vi "Dashboard Main.vi"() -> ()   [LabVIEW 2014]
uses:
  <vilib>/event_ctls.llb/eventvkey.ctl
  <vilib>/Rock Robotics/WPI/Dashboard/WPI_DashboardLogging Global.vi
  <vilib>/Rock Robotics/Network Tables/SD Write Number.vi
  <vilib>/Rock Robotics/Network Tables/SD Write Boolean.vi
  <vilib>/Rock Robotics/Network Tables/SD Read Number.vi
  <vilib>/Rock Robotics/Network Tables/SD Read Boolean.vi
  <vilib>/Rock Robotics/Network Tables/SD Write String.vi
  <vilib>/Utility/config.llb/Write Key (String).vi
  <vilib>/Utility/config.llb/Write Key (I32).vi
  <vilib>/Utility/config.llb/NI_LVConfig.lvlib
panel:
  in  "TCP":refnum<k5>
  in  "Rec Mode":enum32{"Stop", "Record", "Playback"}(radio)
  in  "Vision":u16(ring) items=["Camera Off", "USB Camera SW", "USB Camera HW", "IP Camera"]
  out "Camera IP":string
  out "Image Message":string="Timeout in Camera Communications"
  in  "Dashboard Tab":T1(tab)
  out "Lower Sensor":bool
  out "Middle Sensor":bool
  out "Overide":bool=TRUE
  out "Lift Saftey":bool
  out "Top Sensor":bool
  out "Bottom Sensor":bool
  out "?":bool
  in  "Motor Saftey":bool=TRUE
  in  "Camera Settings":T2={"Frame Rate"=30, "Compression"=30, "Size"=1} {"Frame Rate" scale=1.0..30.0; "Size" items=["640x480", "320x240", "160x120"]}
  out "Gyro":dbl(knob) scale=0.0..360.0
  out "Mode":T3(ring)=enum."Auto Disabled"
  in  "DB Camera Config":bool
  out "fps":dbl format="%#.1g"
  out "Mbps":dbl format="%#.1g"
  out "Mbps 2":bool
  in  "DB/String 9":string
  in  "DB/String 8":string
  in  "DB/String 7":string
  in  "DB/String 6":string
  in  "DB/String 5":string
  in  "DB/String 4":string
  in  "DB/String 3":string
  in  "DB/String 2":string
  in  "DB/String 1":string
  in  "DB/String 0":string
  in  "DB/Slider 0":dbl(slide) scale=0.0..5.0
  in  "DB/Slider 1":dbl(slide) scale=0.0..5.0
  in  "DB/Slider 2":dbl(slide) scale=0.0..5.0
  in  "DB/Slider 3":dbl(slide) scale=0.0..5.0
  out "DB/LED 3":bool
  out "DB/LED 2":bool
  out "DB/LED 1":bool
  out "DB/LED 0":bool
  in  "DB/Button 3":bool
  in  "DB/Button 2":bool
  in  "DB/Button 1":bool
  in  "DB/Button 0":bool caption="New Name"
  in  "Test Slider":dbl(slide) scale=0.0..100.0 scale format="%#_3g"
  in  "On/Off":bool caption="Solenoid"
  in  "Test Name":u16(ring) items=["Select the test to run...", "Example Test", "-------------------------------", "List of tests is built in robot code.", "Replace with your own automated tests."]
  in  "Test Tree":string(tree)
  in  "Motor":cluster{"Value":dbl, "Enable":bool} {"Value" scale=-1.0..1.0 scale format="%#_3g"}
  out "Progress":T4 {"Test Progress" scale=0.0..100.0}
  in  "Rev/Fwd":cluster{"Forward":bool, "Reverse":bool}
  in  "Test Ring":u16(ring) items=["Monochrome", "Color"]
  in  "Listbox":i32(listbox)
  in  "Listbox 2":i32(listbox)=15
  in  "Autonomous Program":i32(listbox)
  in  "Test System Select":enum32{"Motors", "Pneumatics"}(tab)
  in  "Test Motor Mode Select":enum32{"Encoder Mode", "Manual Mode"}(tab)
  in  "?":bool
  in  "Motor Power":dbl(knob) scale=0.0..1.0
  out "?":bool=TRUE
  out "Encoder Feedback":dbl
  in  "Encoder Setpoint":dbl
  out "Encoder RPM":dbl
  in  "?":dbl(knob) scale=-1.0..1.0
  in  "Test Action":string(combo)="Disabled"
  out "?":string="Click the top button to toggle compressor state.\nThe green button indicates if the compressor is running. If the pressure in the system is above 100psi the compressor will turn off."
  out "?":bool
  in  "?":bool
  in  "?":bool
  in  "Solenoid Action":string(combo)="Disabled"
  out "Tree":string(tree)
  out "Camera Image":T5(plugin-control)
  out "Boolean":bool
  # "Top"
  # "Middle"
  # "Lift Saftey"
  # "Lower"
  # "Bottom"
  # "Overide"
  # "This tab is a great place for autonomous settings and robot-specific values.\nPlace controls and indicators inside this tab and match name to\nDashboard Variables on robot. You can also delete this comment."
  # "Select a system to test."
  # "Type in encoder setpoint (Ticks). Then increase the power slowly.  Encoder feedback is the traveled distance.\nThe motor should stop when staus button is green. Press reset to reset encoder."
  # "Simply drag the needle to change motor power. Motor RPM is below."
  # "Pick an action an click the button above. Double acting solenoids are automatically changed."
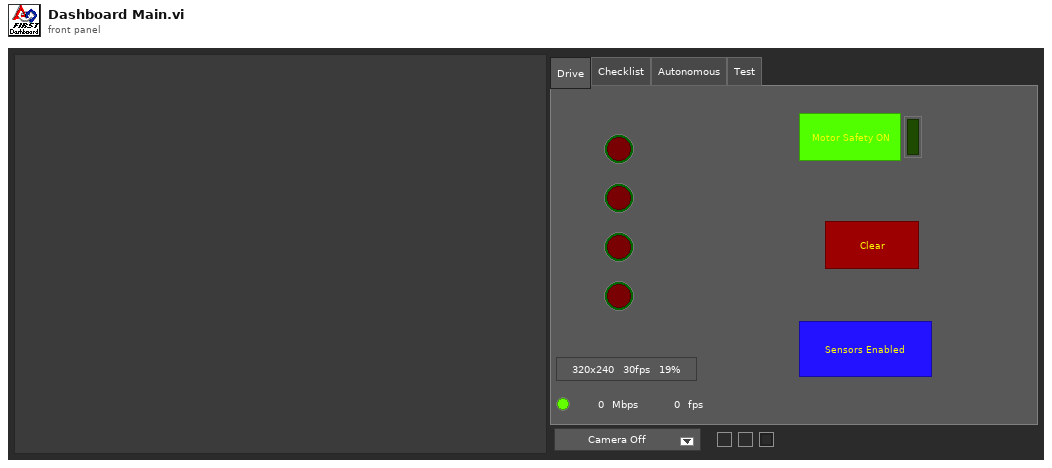
[diagram p1: front panel]
types:
  T1 = enum32{"Drive", "Basic", "Custom", "Test Var", "ChecklistOLD", "Checklist", "Autonomous", "Test", "Variables"}
  T2 = cluster{"Frame Rate":i32, "Compression":i32, "Size":u16}
  T3 = enum8{"Tele-Op Disabled", "Tele-Op Enabled", "Auto Disabled", "Auto Enabled", "Test Disabled", "Test Enabled", "Disconnected", "No Code", "E-Stop"}
  T4 = cluster{"Test Progress":u8, "Test Progress Text":string}
  T5 = typedef "IMAQ Image.ctl" = refnum<image>
  T6 = enum32{"Drive", "Basic", "Custom", "Test", "Checklist", "Variables"}
  T7 = typedef "Image Type" = u32
  T8 = cluster{"Camera Image":refnum<vi>, "Dashboard Tab":refnum<vi>, "Boolean":refnum<vi>, "Vision":refnum<vi>, "Rec Mode":refnum<vi>, "Test Slider":refnum<vi>, "On/Off ":refnum<vi>, "Test Ring":refnum<vi>, "Rev/Fwd":refnum<vi>, "Test Name":refnum<vi>, "Motor":refnum<vi>, "Progress":refnum<vi>, "CheckList":refnum<vi>, "Tree":refnum<vi>, "Test Tree":refnum<vi>}
  T9 = cluster{"Error Strings":string, "Disable Counts":cluster{u16, u16}, "Rail Faults":cluster{u16, u16, u16}, "Robot IP":string, "DB Mode":u8, "Event Info":cluster{"Name":string, "Type":u8, "Number":u16, "Replay":u8}, "Camera Addr":string}
  T10 = cluster{"Storage":cluster{"Disk Free":u64, "RAM Block":u32, "RAM free":u32}, "CPU Utilization":cluster{"CPU % ISR":sgl, "CPU % Time Crit":sgl, "CPU % Timed Str":sgl, "CPU % High":sgl, "CPU % Above":sgl, "CPU % Normal":sgl, "CPU % Low":sgl}, "CAN":cluster{"% Bus Utilization":sgl, "Bus Off Cnt":u32, "TX_FIFO Full Cnt":u32, "Receive Error Cnt":u8, "Transmit Error Cnt":u8}, "HID":cluster{"HID Outputs":u32, "Rumble Low":u16, "Rumble High":u16}[]}
  T11 = cluster{"Status bits":cluster{"Test Mode":bool, "Autonomous":bool, "Enabled":bool, "Code Start":bool, "Brownout":bool, "Reserved 2":bool, "Reserved 3":bool, "E-Stop":bool}, "Code Trace":cluster{"Disabled":bool, "TeleOp":bool, "Auto":bool, "Test":bool}, "Controller Type":enum16{"unknown", "cRIO", "roboRio"}, "Code?":enum16{"unknown", "noCode", "code"}, "Battery V":dbl}
  T12 = cluster{"Control Bits":cluster{"TestMode":bool, "Autonomous":bool, "Enabled":bool, "FMS Present":bool, bool, bool, bool, "E-Stop":bool}, "Team Station ":u8, "Countdown":sgl, "Joystick Values":cluster{"Axes":dbl[], "Buttons":bool[], "POVs":i16[]}[]}
  T13 = typedef "NI_LVConfig.lvlib/Config Data RefNum.ctl" = refnum<k1>
  T14 = cluster{"Operation":enum16{"Update", "Clear"}, "Color Box":u32}[]
  T15 = typedef "eventvkey.ctl" = enum16{"ASCII", "Enter", "Return", "Shift", "Ctrl", "Alt", "Cmd", "Opt", "Caps", "NumLock", "Clear", "Break", "Up", "Down", "Left", "Right", "Insert", "Delete", "Home", "End", "PageUp", "PageDown", "Escape", "Help", "Pause", "ScrollLock", "F1", "F2", "F3", "F4", "F5", "F6", "F7", "F8", "F9", "F10", "F11", "F12", "F13", "F14", "F15", "F16", "F17", "F18", "F19", "F20", "F21", "F22", "F23", "F24", "Play", "VolumeUp", "VolumeDown", "Mute", "Two Byte Char"}
  T16 = cluster{"Image Size":bool, "Image Type":bool, "Pixel Value":bool, "ROI Information":bool, "Zoom Factor":bool}
  T17 = enum8{"Enabled", "Disabled", "Disabled and Grayed Out"}
  T18 = cluster{"Operation":enum16{"Update", "Clear"}, "Color Box":u32}
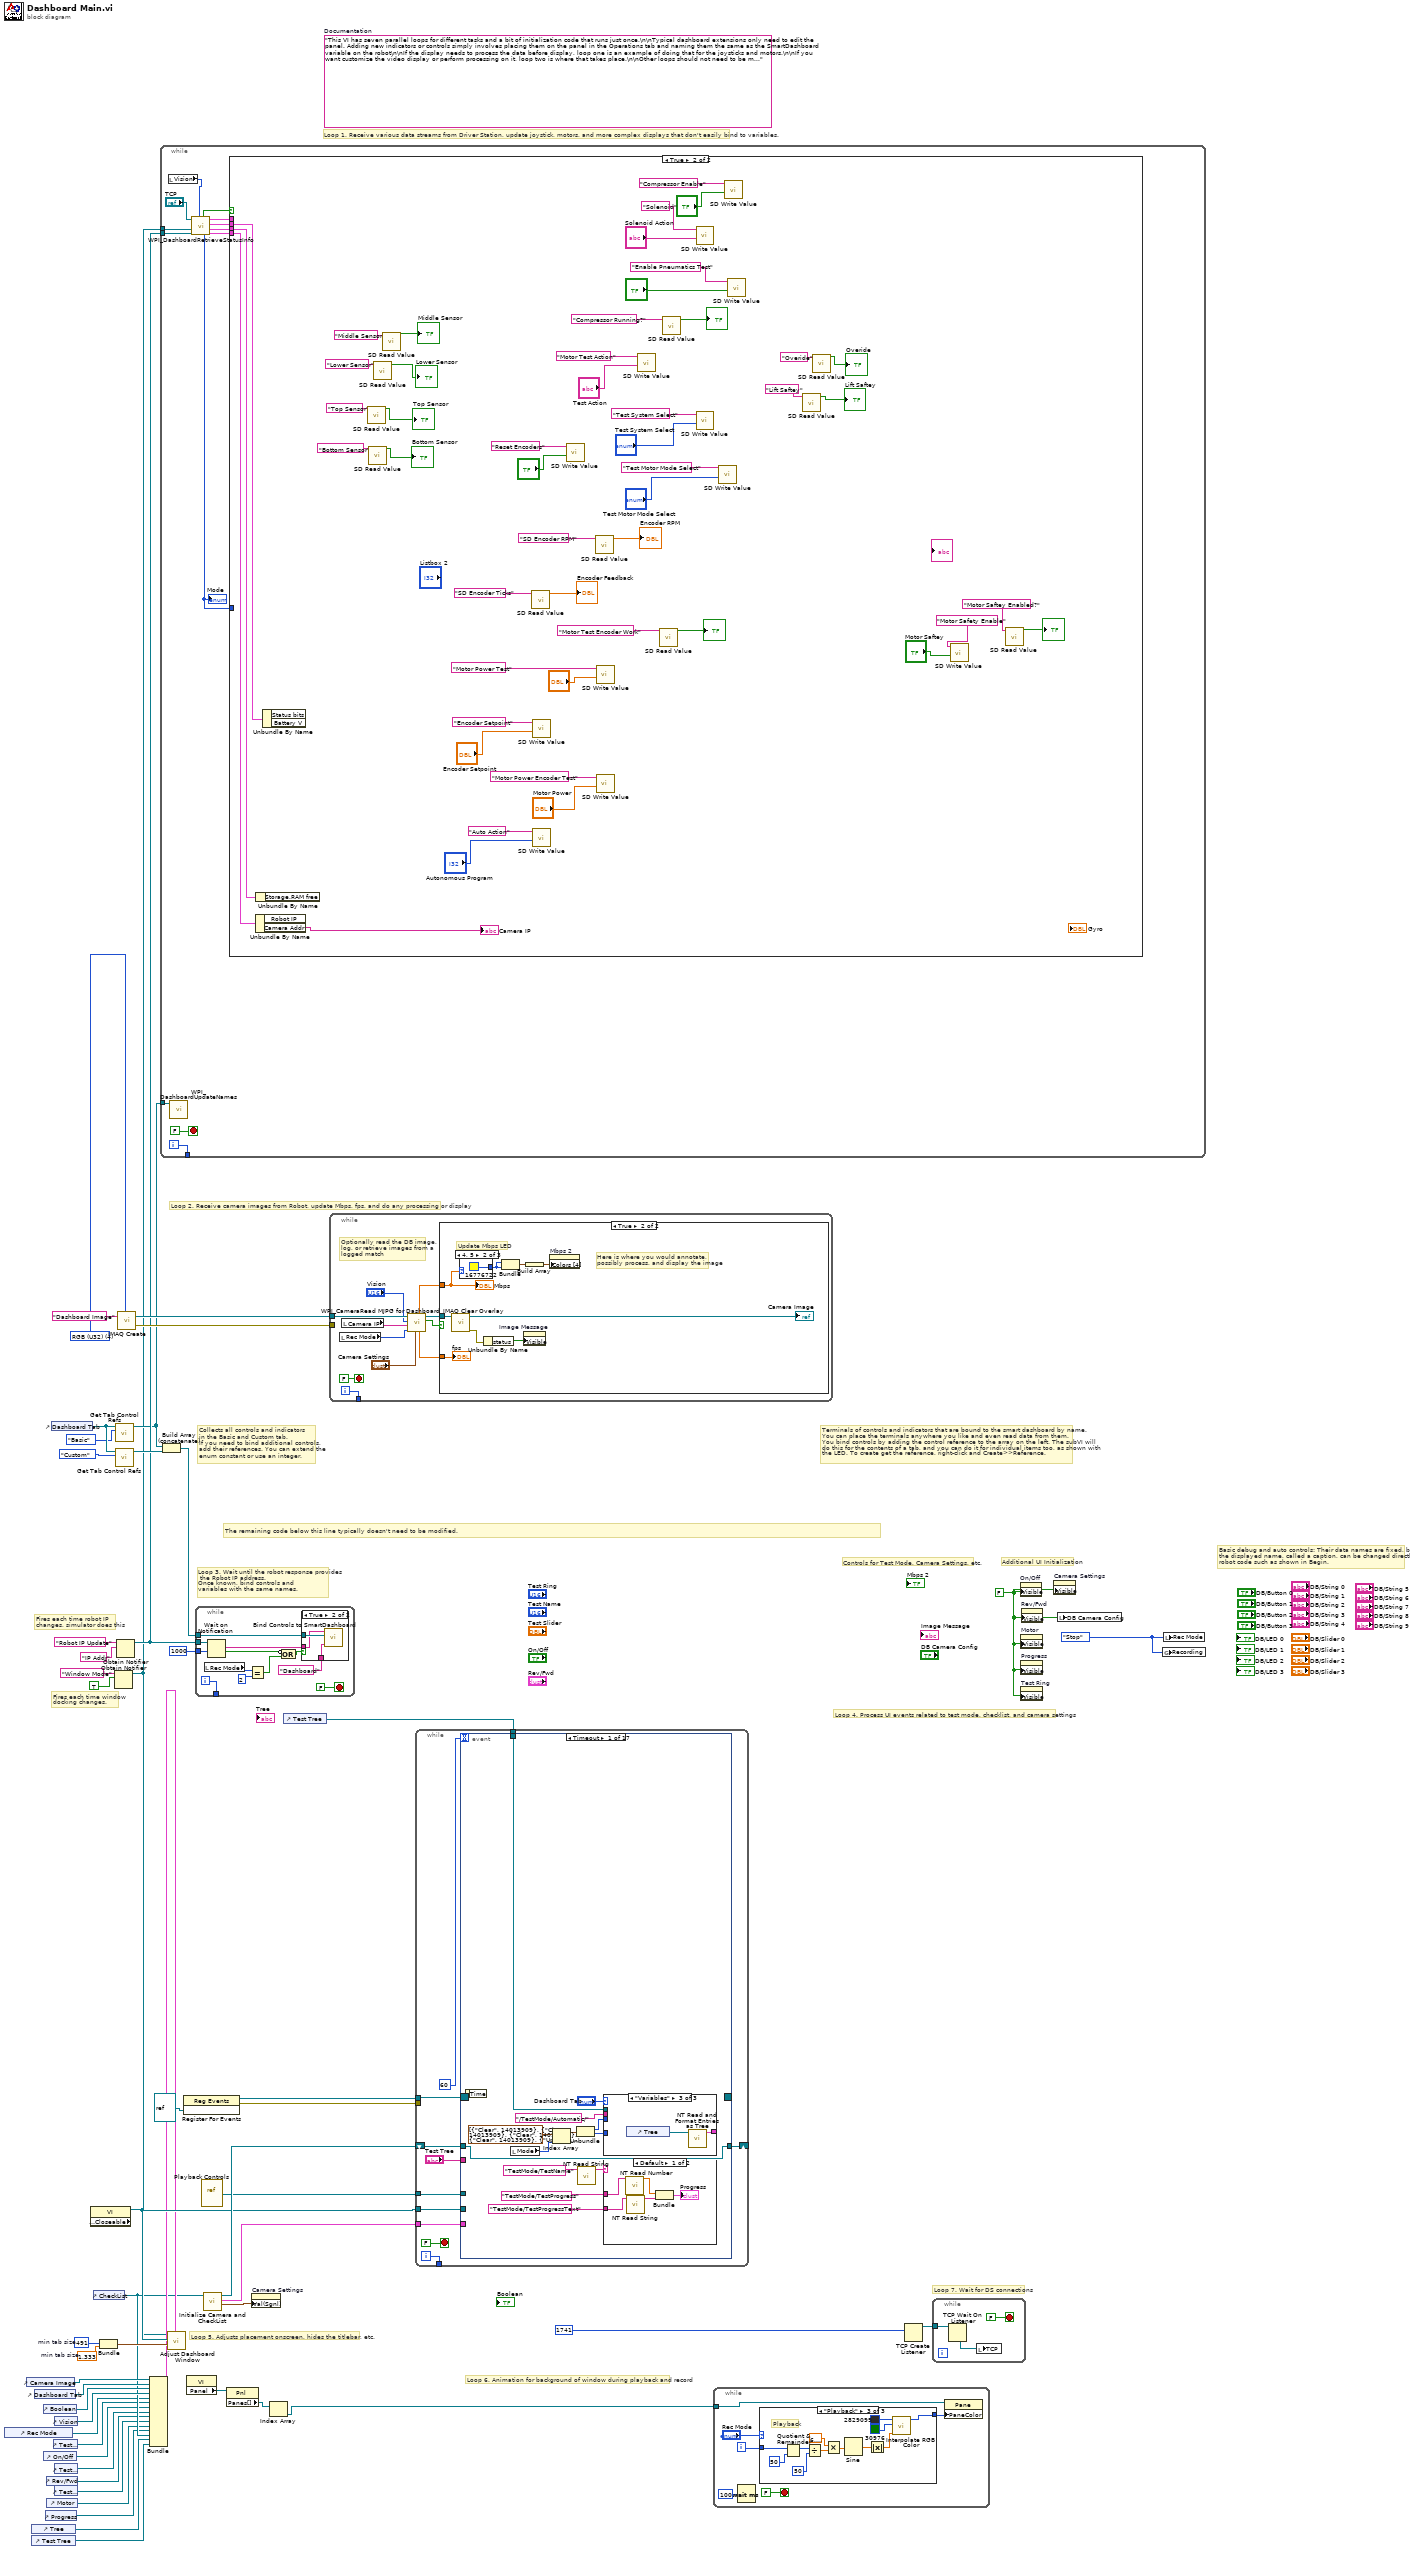
[diagram p0: block diagram]
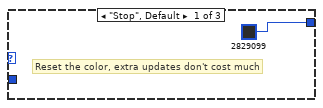
[diagram p3: hidden frame]
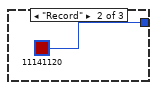
[diagram p4: hidden frame]
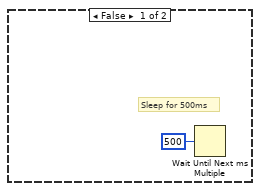
[diagram p6: hidden frame]
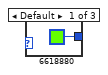
[diagram p7: hidden frame]
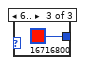
[diagram p8: hidden frame]
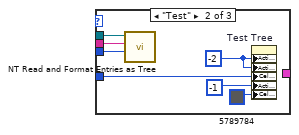
[diagram p10: hidden frame]
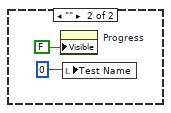
[diagram p11: hidden frame]
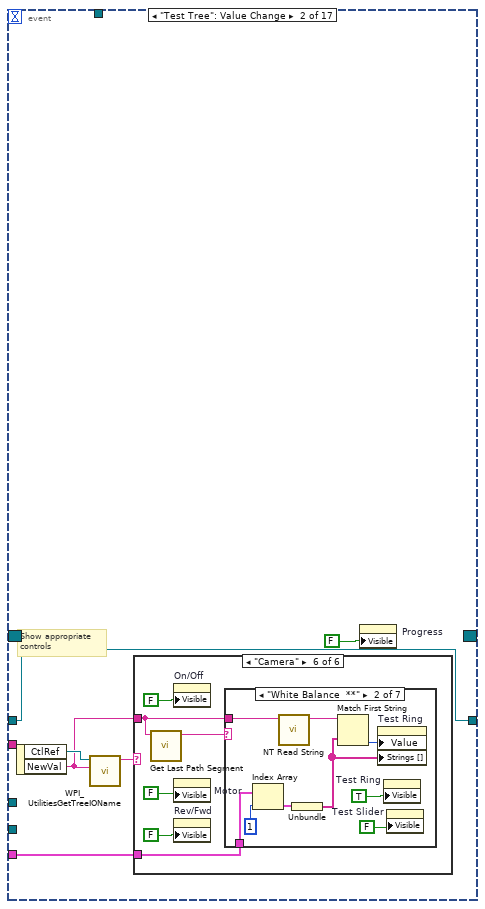
[diagram p12: hidden frame]
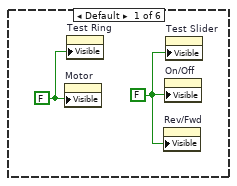
[diagram p13: hidden frame]
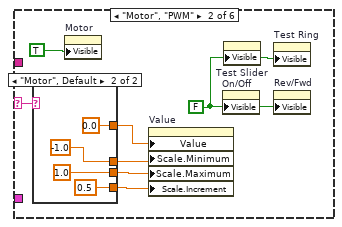
[diagram p14: hidden frame]
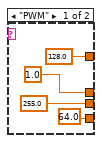
[diagram p15: hidden frame]
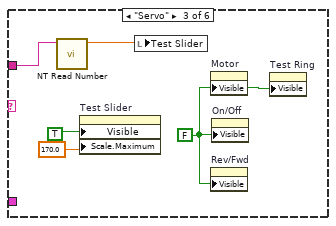
[diagram p16: hidden frame]
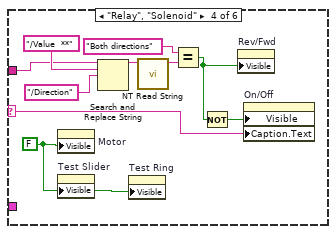
[diagram p17: hidden frame]
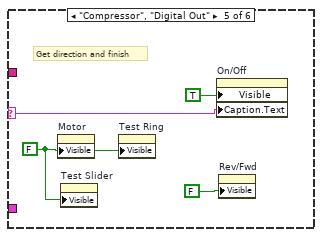
[diagram p18: hidden frame]
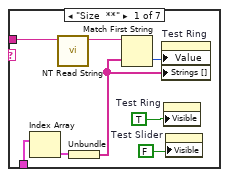
[diagram p19: hidden frame]
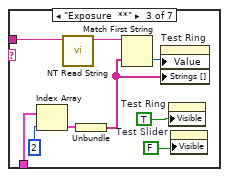
[diagram p20: hidden frame]
diagram:
  w24 = 491  # min tab size
  w23 = 1.333  # min tab size
  w32 = enum32{"Stop", "Record", "Playback"}."Stop" ("Rec Mode")
  w6 = FALSE ("Visible")
  (unwired) "This VI has seven parallel loops for different tasks and a bit of initialization code that runs just once.\n\nTypical dashboard extensions only need to edit the panel. Adding new indicators or controls simply involves placing them on the panel in the Operations tab and naming them the same as the SmartDashboard variable on the robot\n\nIf the display needs to process the data before display, loop one is an example of doing that for the joysticks and motors.\n\nIf you want customize the video display or perform processing on it, loop two is where that takes place.\n\nOther loops should not need to be modified. They are pretty standard, and document the task they perform."  # Documentation
  w52 = T7 4 items=["Grayscale (U8)", "Grayscale (I16)", "Grayscale (SGL)", "Complex (CSG)", "RGB (U32)", "HSL (U32)", "RGB (U64)"] ("Image Type")
  # "Loop 7. Wait for DS connections"
  # "Basic debug and auto controls: Their data names are fixed, but\nthe displayed name, called a caption, can be changed directly or in\nrobot code such as shown in Begin."
  # "Controls for Test Mode, Camera Settings, etc."
  # "Additional UI Initialization"
  # "Loop 6. Animation for background of window during playback and record"
  # "Fires each time robot IP\nchanges, simulator does this"
  # "Fires each time window\ndocking changes."
  # "Collects all controls and indicators\nin the Basic and Custom tab.\nIf you need to bind additional controls,\nadd their references. You can extend the\nenum constant or use an integer."
  # "The remaining code below this line typically doesn't need to be modified."
  # "Loop 4. Process UI events related to test mode, checklist, and camera settings"
  # "Terminals of controls and indicators that are bound to the smart dashboard by name.\nYou can place the terminals anywhere you like and even read data from them.\nYou bind controls by adding the control reference to the array on the left. The subVI will\ndo this for the contents of a tab, and you can do it for individual items too, as shown with\nthe LED. To create get the reference, right-click and Create>>Reference."
  # "Loop 3. Wait until the robot response provides\n the Robot IP address.\nOnce known, bind controls and\nvariables with the same names."
  # "Loop 5. Adjusts placement onscreen, hides the titlebar, etc."
  # "Loop 1. Receive various data streams from Driver Station, update joystick, motors, and more complex displays that don't easily bind to variables."
  # "Loop 2. Receive camera images from Robot, update Mbps, fps, and do any processing or display"
  n1 = control-ref of="Rec Mode"() -> (w12:refnum<vi>)
  n2 = control-ref of="Camera Image"() -> (w27:refnum<vi>)
  n3 = control-ref of="Tree"() -> (w16:refnum<vi>)
  n4 = control-ref of="Test Tree"() -> (w15:refnum<vi>)
  n5 = control-ref of="Dashboard Tab"() -> (w26:refnum<vi>)
  n6 = control-ref of="Boolean"() -> (w21:refnum<vi>)
  n7 = control-ref of="On/Off"() -> (w10:refnum<vi>)
  n8 = control-ref of="Progress"() -> (w7:refnum<vi>)
  n9 = control-ref of="Rev/Fwd"() -> (w8:refnum<vi>)
  n10 = control-ref of="Motor"() -> (w13:refnum<vi>)
  n11 = control-ref of="Dashboard Tab"() -> (w30:refnum<vi>)
  n12 = control-ref of="Test Slider"() -> (w11:refnum<vi>)
  n13 = control-ref of="Vision"() -> (w25:refnum<vi>)
  n14 = control-ref of="Test Ring"() -> (w9:refnum<vi>)
  n15 = control-ref of="Test Name"() -> (w14:refnum<vi>)
  n16 = property class="VI" props=["Front Panel.Closeable"]() -> (reference out=w31:refnum<vi>)  [unwired: 2 in, 2 out]
  n17 = control-ref of="CheckList"() -> (w17:refnum<vi>)
  n18 = Bundle("min tab size"=w24, "min tab size"=w23) -> (w22:cluster{"min tab size":i32, "min tab size":dbl})  [unwired: 1 in]
  n19 = Obtain Notifier(name (unnamed)="Window Mode", notification data type=TRUE) -> (notifier out=w3:refnum<notifier>)  [unwired: 2 in, 2 out]
  n20 = call <vilib>:"Get Tab Control Refs.vi"("Page Index"=T6."Basic" ("Dashboard Tab"), "TabControl in"=w30) -> ("ControlsOnPage"=w4:refnum<vi>[])  [unwired: 9 in]
  n21 = call <vilib>:"Get Tab Control Refs.vi"("Page Index"=T6."Custom" ("Dashboard Tab"), "TabControl in"=w30) -> ("ControlsOnPage"=w29:refnum<vi>[])  [unwired: 9 in]
  n22 = Obtain Notifier(name (unnamed)="Robot IP Update", notification data type="IP Addr" ("name (unnamed)")) -> (notifier out=w5:refnum<notifier>)  [unwired: 2 in, 2 out]
  n23 = call "IMAQ Create"("Image Name"="Dashboard Image", "Image Type"=w52) -> ("New Image"=w50:T5, "error out"=w49:errorcluster)  [unwired: 2 in, 1 out]
  n24 = Bundle("Camera Image"=w27, "Dashboard Tab"=w26, "Boolean"=w21, "Vision"=w25, "Rec Mode"=w12, "Test Slider"=w11, "On/Off"=w10, "Test Ring"=w9, "Rev/Fwd"=w8, "Test Name"=w14, "Motor"=w13, "Progress"=w7, "CheckList"=w17, "Tree"=w16, "Test Tree"=w15) -> (w18:T8)  [unwired: 1 in]
  n25 = while {
    tunnel: [w64] -> _
    tunnel: w5 -> [w58]
    tunnel: w4 -> [w57]
    tunnel: w3 -> [w53]
    i -> [w64]
    stop <- FALSE stop-if-true
    n26 = local read "Vision"() -> (w55:u16)
    n27 = call <vilib>:"WPI_DashboardUpdateNames.vi"("Controls on Tab"=w57) -> ()  [unwired: 11 in]
    n28 = call <vilib>:"WPI_DashboardRetrieveStatusInfo.vi"("Vision"=w55, "Binding Refnum"=w58, "Window Mode Notifier"=w53, "TCP Cnx"="TCP") -> ("Power and Errors"=w59:T9, "Robot Metrics"=w62:T10, "Status Info"=w63:T11, "Control Info"=w60:T12, "Robot Mode"=w56:T3, "Process?"=w61:bool)  [unwired: 2 in]
    "Mode" <- w56
    n29 = case shown="True" w61 {
      tunnel: w63 -> [_ w115]
      tunnel: w62 -> [_ w114]
      tunnel: w60 -> [_ _]
      tunnel: w59 -> [_ w113]
      tunnel: w56 -> [_ _]
      frame False {
      }
      frame True {
        n30 = Unbundle By Name(w113) -> ("Camera Addr"=→"Camera IP":string)  [unwired: 1 out]
        n31 = Unbundle By Name(w114) -> ()  [unwired: 1 out]
        n32 = Unbundle By Name(w115) -> ()  [unwired: 2 out]
        n33 = call-poly <vilib>:"SD Read Value.vi"("Name"="Top Sensor") -> ("Boolean"=→"Top Sensor":bool)  [unwired: 8 in, 2 out]
        n34 = call-poly <vilib>:"SD Read Value.vi"("Name"="Bottom Sensor") -> ("Boolean"=→"Bottom Sensor":bool)  [unwired: 8 in, 2 out]
        n35 = call-poly <vilib>:"SD Read Value.vi"("Name"="Lower Sensor") -> ("Boolean"=→"Lower Sensor":bool)  [unwired: 8 in, 2 out]
        n36 = call-poly <vilib>:"SD Read Value.vi"("Name"="Middle Sensor") -> ("Boolean"=→"Middle Sensor":bool)  [unwired: 8 in, 2 out]
        n37 = call-poly <vilib>:"SD Read Value.vi"("Name"="SD Encoder Ticks") -> ("Numeric"=→"Encoder Feedback":dbl)  [unwired: 8 in, 2 out]
        n38 = call-poly <vilib>:"SD Write Value.vi"("Numeric"="Encoder Setpoint", "Name"="Encoder Setpoint") -> ()  [unwired: 8 in, 2 out]
        n39 = call-poly <vilib>:"SD Write Value.vi"("Numeric"="Autonomous Program", "Name"="Auto Action") -> ()  [unwired: 8 in, 2 out]
        n40 = call-poly <vilib>:"SD Write Value.vi"("Boolean"="?", "Name"="Reset Encoders") -> ()  [unwired: 8 in, 2 out]
        n41 = call-poly <vilib>:"SD Read Value.vi"("Name"="SD Encoder RPM") -> ("Numeric"=→"Encoder RPM":dbl)  [unwired: 8 in, 2 out]
        n42 = call-poly <vilib>:"SD Write Value.vi"("Numeric"="?", "Name"="Motor Power Test") -> ()  [unwired: 8 in, 2 out]
        n43 = call-poly <vilib>:"SD Write Value.vi"("Numeric"="Motor Power", "Name"="Motor Power Encoder Test") -> ()  [unwired: 8 in, 2 out]
        n44 = call-poly <vilib>:"SD Write Value.vi"("String"="Test Action", "Name"="Motor Test Action") -> ()  [unwired: 8 in, 2 out]
        n45 = call-poly <vilib>:"SD Read Value.vi"("Name"="Motor Test Encoder Work") -> ("Boolean"=→"?":bool)  [unwired: 8 in, 2 out]
        n46 = call-poly <vilib>:"SD Read Value.vi"("Name"="Compressor Running?") -> ("Boolean"=→"?":bool)  [unwired: 8 in, 2 out]
        n47 = call-poly <vilib>:"SD Write Value.vi"("String"="Solenoid Action", "Name"="Solenoid") -> ()  [unwired: 8 in, 2 out]
        n48 = call-poly <vilib>:"SD Write Value.vi"("Numeric"="Test System Select", "Name"="Test System Select") -> ()  [unwired: 8 in, 2 out]
        n49 = call-poly <vilib>:"SD Write Value.vi"("Numeric"="Test Motor Mode Select", "Name"="Test Motor Mode Select") -> ()  [unwired: 8 in, 2 out]
        n50 = call-poly <vilib>:"SD Write Value.vi"("Boolean"="?", "Name"="Compressor Enable") -> ()  [unwired: 8 in, 2 out]
        n51 = call-poly <vilib>:"SD Write Value.vi"("Boolean"="?", "Name"="Enable Pneumatics Test") -> ()  [unwired: 8 in, 2 out]
        n52 = call-poly <vilib>:"SD Read Value.vi"("Name"="Lift Saftey") -> ("Boolean"=→"Lift Saftey":bool)  [unwired: 8 in, 2 out]
        n53 = call-poly <vilib>:"SD Read Value.vi"("Name"="Overide") -> ("Boolean"=→"Overide":bool)  [unwired: 8 in, 2 out]
        n54 = call-poly <vilib>:"SD Write Value.vi"("Boolean"="Motor Saftey", "Name"="Motor Safety Enable") -> ()  [unwired: 8 in, 2 out]
        n55 = call-poly <vilib>:"SD Read Value.vi"("Name"="Motor Saftey Enabled?") -> ("Boolean"=→"?":bool)  [unwired: 8 in, 2 out]
      }
    }
  }
  n56 = Build Array (concatenate)(w4, w29) -> (w28:refnum<vi>[])
  n57 = call "Adjust Dashboard Window.vi"("Sizing Refnums"=w18, "Size Constraints"=w22, "VI"=w31, "Notifier in"=w3) -> ()  [unwired: 8 in]
  n58 = register-events(refnum<vi> refnum) -> (reference out=w36:refnum<event-registration>, error out=w35:errorcluster)  [unwired: 2 in]
  n59 = property class="VI"() -> ("Panel"=w39:refnum<vi>)  [unwired: 2 in, 2 out]
  n60 = while {
    tunnel: w28 -> [w127]
    tunnel: w5 -> [w125]
    tunnel: [w123] -> _
    tunnel: u32 1000 ("milliseconds to wait") -> [w122]
    i -> [w123]
    stop <- FALSE stop-if-true
    n61 = local read "Rec Mode"() -> (w118:enum32{"Stop", "Record", "Playback"})
    n62 = Wait on Notification(notifier=w125, timeout in ms (-1)=w122) -> (notification=w124:string, timed out?=w120:bool)  [unwired: 2 in, 2 out]
    n63 = Equal?(x=w118, y=u16 2 ("Rec Mode")) -> (x = y?=w119:bool)
    n64 = Compound Arithmetic op=OR(invert w120, w119) -> (w121:bool)
    n65 = case shown="True" w121 {
      tunnel: w127 -> [_ w130]
      tunnel: w124 -> [_ w129]
      tunnel: "Dashboard" -> [_ w128]
      frame False {
      }
      frame True {
        n66 = call <vilib>:"Bind Controls to SmartDashboard.vi"("Client Name"=w128, "Bound Control Refs"=w130, "Server IP Address"=w129) -> ()  [unwired: 9 in]
      }
    }
  }
  n67 = vi-ref "Playback Controls.vi"() -> (w37:refnum<vi>)
  n68 = call "Initialize Camera and CheckList.vi"("ListBox in"=w17) -> ("Cluster"=w43:cluster{"value":i32, "value":i32, "index":i32}, "Array"=w44:cluster{string[]}[], "File Refnum"=w42:T13)  [unwired: 8 in]
  n69 = property class="Pnl"(reference=w39) -> ("Panes[]"=w40:refnum<vi>[])  [unwired: 1 in, 2 out]
  n70 = property on="Camera Settings" class="Clust (strict)"("Val(Sgnl)"=w43) -> ()  [unwired: 2 in, 2 out]
  n71 = Index Array(array=w40) -> (element=w38:refnum<vi>)  [unwired: 1 in]
  n72 = control-ref of="Test Tree"() -> (w41:refnum<vi>)
  n73 = while {
    tunnel: w50 -> [w139]
    tunnel: w49 -> [_]
    tunnel: [w140] -> _
    i -> [w140]
    stop <- FALSE stop-if-true
    # "Optionally read the DB image,\nlog, or retrieve images from a\nlogged match"
    n74 = local read "Rec Mode"() -> (w133:enum32{"Stop", "Record", "Playback"})
    n75 = local read "Camera IP"() -> (w131:string)
    n76 = call <vilib>:"WPI_CameraRead MJPG for Dashboard.vi"("Camera Settings"="Camera Settings", "Rec Mode"=w133, "Camera IP"=w131, "Camera Mode"="Vision", "Refnum in"=w139) -> ("Active"=w137:bool, "Refnum out"=w138:T5, "FPS"=w136:dbl, "Bandwidth (Mbps)"=w135:dbl)  [unwired: 3 in]
    n77 = case shown="True" w137 {
      tunnel: w138 -> [_ w146]
      tunnel: w135 -> [_ w145]
      tunnel: w136 -> [_ w143]
      frame False {
        # "Sleep for 500ms"
        n78 = Wait Until Next ms Multiple(millisecond multiple=u32 500) -> ()  [unwired: 1 out]
      }
      frame True {
        # "Here is where you would annotate,\npossibly process, and display the image"
        # "Update Mbps LED"
        n79 = call "IMAQ Clear Overlay"("Image"=w146) -> ("error out"=w150:errorcluster, "Image Out"=→"Camera Image":T5)  [unwired: 2 in, 7 out]
        n80 = case shown="4, 5" w145 {
          tunnel: [u32 6618880 ("Color Box") u32 16776722 ("Color Box") u32 16716800 ("Color Box")] -> w147
          frame Default {
          }
          frame 4, 5 {
          }
          frame 6.. {
          }
        }
        n81 = Unbundle By Name(w150) -> ("status"=w151:bool)
        n82 = Bundle("Color Box"=w147, "Color Box"=w147) -> (w149:cluster{"Color Box":u32, "Color Box":u32})  [unwired: 1 out]
        n83 = property on="Image Message" class="Str"("Visible"=w151) -> ()  [unwired: 2 in, 2 out]
        n84 = Build Array(w149) -> (w148:cluster{"Color Box":u32, "Color Box":u32}[])
        n85 = property on="Mbps 2" class="Bool (strict)"("Colors [4]"=w148) -> ()  [unwired: 2 in, 2 out]
        "Mbps" <- w145
        "fps" <- w143
      }
    }
  }
  n86 = while {
    tunnel: w44 -> [w162]
    shift-right: [w161] -> _
    shift-left: w42 -> [w160]
    tunnel: [w159] -> _
    tunnel: w41 -> [w158]
    tunnel: w37 -> [w157]
    tunnel: w36 -> [w156]
    tunnel: w35 -> [_]
    tunnel: w31 -> [w155]
    i -> [w159]
    stop <- FALSE stop-if-true
    n87 = event shown="[0] Timeout" {
      selector: w156 -> [_ _ _ _ _ _ _ _ _ _ _ _ _ _ _ _ _]
      dyn-events: [_ _ _ _ _ _ _ _ _ _ _ _ _ w400 _ _ _] -> _
      timeout: u32 60 ("milliseconds to wait") -> [_ _ _ _ _ _ _ _ _ _ _ _ _ _ _ _ _]
      tunnel: w158 -> [w174 _ _ _ _ _ _ _ _ _ _ _ _ _ _ _ _]
      tunnel: "Test Tree" -> [_ _ _ _ _ _ _ _ w369 w377 w379 w383 w391 _ _ _ _]
      tunnel: w162 -> [_ w196 _ _ _ _ w333 w363 _ _ _ _ _ _ _ _ _]
      tunnel: [w170 w195 w294 w299 w307 w319 w332 w356 w368 w375 w378 w382 w390 w402 w416 w417 w427] -> w161
      tunnel: w160 -> [w170 w195 w294 w299 w307 w319 w331 w356 w368 w375 w378 w382 w390 w402 w416 w417 w427]
      tunnel: w157 -> [_ _ _ _ _ _ _ _ _ _ _ _ _ w403 _ w420 _]
      tunnel: w155 -> [_ _ _ _ _ _ _ _ _ _ _ _ _ w398 _ _ _]
      event Timeout {
        n88 = event-data() -> ()  [unwired: 1 in, 1 out]
        n89 = local read "Mode"() -> (w173:T3)
        n90 = Index Array(array=T14 [{"Operation"=enum."Clear", "Color Box"=14013909}, {"Operation"=enum."Clear", "Color Box"=14013909}, {"Operation"=enum."Clear", "Color Box"=14013909}, {"Operation"=enum."Clear", "Color Box"=14013909}, {"Operation"=enum."Update", "Color Box"=14013909}, {"Operation"=enum."Update", "Color Box"=16777215}, {"Operation"=enum."Clear", "Color Box"=14013909}, {"Operation"=enum."Clear", "Color Box"=14013909}, {"Operation"=enum."Clear", "Color Box"=14013909}], index=w173) -> (element=w168:T18)
        n91 = Unbundle(w168) -> ("Operation"=w167:enum16{"Update", "Clear"}, "Color Box"=w166:u32)
        n92 = call <vilib>:"NT Read String.vi"("Name"="TestMode/TestName") -> ("String"=w177:string)  [unwired: 9 in, 1 out]
        n93 = case shown="\"Variables\"" "Dashboard Tab" {
          tunnel: w174 -> [_ w185 _]
          tunnel: "/TestMode/Automatic/" ("Name Pattern") -> [_ w184 _]
          tunnel: w167 -> [_ w183 _]
          tunnel: [_ _ w187] -> _
          tunnel: w166 -> [_ w179 _]
          frame "Custom", Default {
          }
          frame "Test" {
            w182 = -2 ("Active Item:Row Number")
            n94 = call <vilib>:"NT Read and Format Entries as Tree.vi"("Operation"=w183, "Name Pattern"=w184, "Tree Refnum"=w185) -> ()  [unwired: 7 in, 2 out]
            n95 = property on="Test Tree" class="Tree (strict)"("Active Item Row Number"=w182, "ActiveColNum"=w182, "CellBG"=w179, "Active Item Row Number"=-1 ("Active Item:Row Number"), "CellBG"=u32 5789784 ("Color Box")) -> ()  [unwired: 2 in, 2 out]
          }
          frame "Variables" {
            n96 = control-ref of="Tree"() -> (w186:refnum<vi>)
            n97 = call <vilib>:"NT Read and Format Entries as Tree.vi"("Tree Refnum"=w186) -> ("Formatted Strings"=w187:cluster{"Name":string, "Value":string}[])  [unwired: 9 in, 1 out]
          }
        }
        n98 = case shown="Default" w177 {
          tunnel: "TestMode/TestProgress" ("Name") -> [w189 _]
          tunnel: "TestMode/TestProgressText" ("Name") -> [w188 _]
          frame Default {
            n99 = call <vilib>:"NT Read Number.vi"("Name"=w189) -> ("Numeric"=w190:dbl)  [unwired: 9 in, 1 out]
            n100 = call <vilib>:"NT Read String.vi"("Name"=w188) -> ("String"=w191:string)  [unwired: 9 in, 1 out]
            n101 = Bundle("Numeric"=w190, "String"=w191) -> (→"Progress":cluster{"Numeric":dbl, "String":string})  [unwired: 1 in]
          }
          frame "" {
            n102 = property on="Progress" class="Clust (strict)"("Visible"=FALSE) -> ()  [unwired: 2 in, 2 out]
            n103 = local write "Test Name"(u16 0) -> ()
          }
        }
      }
      event "Test Tree": Value Change {
        # "Show appropriate\ncontrols"
        n104 = event-data() -> ("CtlRef"=w199:refnum<vi>, "NewVal"=w197:string)  [unwired: 1 in]
        n105 = call <vilib>:"WPI_UtilitiesGetTreeIOName.vi"("NewVal"=w197, "TreeControl in"=w199) -> ("I/O Name"=w200:string)  [unwired: 9 in]
        n106 = case shown="\"Camera\"" w200 {
          selector: w200 -> [_ w207 _ w225 w234 _]
          tunnel: w197 -> [_ _ w222 w224 _ w241]
          tunnel: w196 -> [_ _ _ _ _ w240]
          frame Default {
            w202 = FALSE ("Visible")
            w201 = FALSE ("Visible")
            n107 = property on="Motor" class="Clust (strict)"("Visible"=w201) -> ()  [unwired: 2 in, 2 out]
            n108 = property on="Test Ring" class="Ring (strict)"("Visible"=w201) -> ()  [unwired: 2 in, 2 out]
            n109 = property on="Rev/Fwd" class="Clust (strict)"("Visible"=w202) -> ()  [unwired: 2 in, 2 out]
            n110 = property on="On/Off" class="Bool (strict)"("Visible"=w202) -> ()  [unwired: 2 in, 2 out]
            n111 = property on="Test Slider" class="Slide (strict)"("Visible"=w202) -> ()  [unwired: 2 in, 2 out]
          }
          frame "Motor", "PWM" {
            w208 = FALSE ("Visible")
            n112 = case shown="\"Motor\", Default" w207 {
              tunnel: [1.0 ("Value") -1.0 ("Value")] -> w206
              tunnel: [255.0 ("Value") 1.0 ("Value")] -> w205
              tunnel: [128.0 ("Value") 0.0 ("Value")] -> w204
              tunnel: [64.0 ("Value") 0.5 ("Value")] -> w203
              frame "PWM" {
              }
              frame "Motor", Default {
              }
            }
            n113 = property on="Motor" class="Clust (strict)"("Visible"=TRUE) -> ()  [unwired: 2 in, 2 out]
            n114 = property on="Value" class="Slide (strict)"("Value"=w204, "Scale.Minimum"=w206, "Scale.Maximum"=w205, "Scale.Increment"=w203) -> ()  [unwired: 2 in, 2 out]
            n115 = property on="On/Off" class="Bool (strict)"("Visible"=w208) -> ()  [unwired: 2 in, 2 out]
            n116 = property on="Test Slider" class="Slide (strict)"("Visible"=w208) -> ()  [unwired: 2 in, 2 out]
            n117 = property on="Test Ring" class="Ring (strict)"("Visible"=w208) -> ()  [unwired: 2 in, 2 out]
            n118 = property on="Rev/Fwd" class="Clust (strict)"("Visible"=w208) -> ()  [unwired: 2 in, 2 out]
          }
          frame "Servo" {
            w220 = FALSE ("Visible")
            n119 = call <vilib>:"NT Read Number.vi"("Name"=w222) -> ("Numeric"=w221:dbl)  [unwired: 9 in, 1 out]
            n120 = property on="Test Slider" class="Slide (strict)"("Visible"=TRUE, "Scale.Maximum"=170.0 ("Scale.Range:Maximum")) -> ()  [unwired: 2 in, 2 out]
            n121 = local write "Test Slider"(w221) -> ()
            n122 = property on="Motor" class="Clust (strict)"("Visible"=w220) -> ()  [unwired: 2 in, 2 out]
            n123 = property on="Rev/Fwd" class="Clust (strict)"("Visible"=w220) -> ()  [unwired: 2 in, 2 out]
            n124 = property on="On/Off" class="Bool (strict)"("Visible"=w220) -> ()  [unwired: 2 in, 2 out]
            n125 = property on="Test Ring" class="Ring (strict)"("Visible"=w220) -> ()  [unwired: 2 in, 2 out]
          }
          frame "Relay", "Solenoid" {
            w223 = FALSE ("Visible")
            n126 = property on="Motor" class="Clust (strict)"("Visible"=w223) -> ()  [unwired: 2 in, 2 out]
            n127 = property on="Test Slider" class="Slide (strict)"("Visible"=w223) -> ()  [unwired: 2 in, 2 out]
            n128 = Search and Replace String(input string=w224, search string="/Value  **", replace string="/Direction") -> (result string=w230:string)  [unwired: 5 in, 3 out]
            n129 = property on="Test Ring" class="Ring (strict)"("Visible"=w223) -> ()  [unwired: 2 in, 2 out]
            n130 = call <vilib>:"NT Read String.vi"("Name"=w230) -> ("String"=w228:string)  [unwired: 9 in, 1 out]
            n131 = Equal?(x="Both directions", y=w228) -> (x = y?=w226:bool)
            n132 = Not(x=w226) -> (.not. x?=w227:bool)
            n133 = property on="Rev/Fwd" class="Clust (strict)"("Visible"=w226) -> ()  [unwired: 2 in, 2 out]
            n134 = property on="On/Off" class="Bool (strict)"("Visible"=w227, "Caption.Text"=w225) -> ()  [unwired: 2 in, 2 out]
          }
          frame "Compressor", "Digital Out" {
            w233 = FALSE ("Visible")
            # "Get direction and finish"
            n135 = property on="Motor" class="Clust (strict)"("Visible"=w233) -> ()  [unwired: 2 in, 2 out]
            n136 = property on="Test Slider" class="Slide (strict)"("Visible"=w233) -> ()  [unwired: 2 in, 2 out]
            n137 = property on="Test Ring" class="Ring (strict)"("Visible"=w233) -> ()  [unwired: 2 in, 2 out]
            n138 = property on="On/Off" class="Bool (strict)"("Visible"=TRUE, "Caption.Text"=w234) -> ()  [unwired: 2 in, 2 out]
            n139 = property on="Rev/Fwd" class="Clust (strict)"("Visible"=FALSE) -> ()  [unwired: 2 in, 2 out]
          }
          frame "Camera" {
            n140 = call <vilib>:"Get Last Path Segment.vi"("String in"=w241) -> ("String out"=w242:string)  [unwired: 10 in]
            n141 = property on="On/Off" class="Bool (strict)"("Visible"=FALSE) -> ()  [unwired: 2 in, 2 out]
            n142 = property on="Motor" class="Clust (strict)"("Visible"=FALSE) -> ()  [unwired: 2 in, 2 out]
            n143 = property on="Rev/Fwd" class="Clust (strict)"("Visible"=FALSE) -> ()  [unwired: 2 in, 2 out]
            n144 = case shown="\"White Balance  **\"" w242 {
              tunnel: w241 -> [w248 w257 w266 w275 w284 _ w290]
              tunnel: w240 -> [w246 w254 w263 w272 w281 _ _]
              frame "Size  **" {
                n145 = Index Array(array=w246) -> (element=w245:cluster{string[]})  [unwired: 1 in]
                n146 = call <vilib>:"NT Read String.vi"("Name"=w248) -> ("String"=w247:string)  [unwired: 9 in, 1 out]
                n147 = Unbundle(w245) -> (w243:string[])
                n148 = Match First String(2:w243, 3:w247) -> (0:w244:i32)  [unwired: 1 out]
                n149 = property on="Test Ring" class="Ring (strict)"("Value"=w244, "Strings []"=w243) -> ()  [unwired: 2 in, 2 out]
                n150 = property on="Test Ring" class="Ring (strict)"("Visible"=TRUE) -> ()  [unwired: 2 in, 2 out]
                n151 = property on="Test Slider" class="Slide (strict)"("Visible"=FALSE) -> ()  [unwired: 2 in, 2 out]
              }
              frame "White Balance  **" {
                n152 = Index Array(array=w254, index=1) -> (element=w255:cluster{string[]})
                n153 = call <vilib>:"NT Read String.vi"("Name"=w257) -> ("String"=w256:string)  [unwired: 9 in, 1 out]
                n154 = Unbundle(w255) -> (w252:string[])
                n155 = Match First String(2:w252, 3:w256) -> (0:w251:i32)  [unwired: 1 out]
                n156 = property on="Test Ring" class="Ring (strict)"("Value"=w251, "Strings []"=w252) -> ()  [unwired: 2 in, 2 out]
                n157 = property on="Test Ring" class="Ring (strict)"("Visible"=TRUE) -> ()  [unwired: 2 in, 2 out]
                n158 = property on="Test Slider" class="Slide (strict)"("Visible"=FALSE) -> ()  [unwired: 2 in, 2 out]
              }
              frame "Exposure  **" {
                n159 = Index Array(array=w263, index=2) -> (element=w264:cluster{string[]})
                n160 = call <vilib>:"NT Read String.vi"("Name"=w266) -> ("String"=w265:string)  [unwired: 9 in, 1 out]
                n161 = Unbundle(w264) -> (w260:string[])
                n162 = Match First String(2:w260, 3:w265) -> (0:w261:i32)  [unwired: 1 out]
                n163 = property on="Test Ring" class="Ring (strict)"("Value"=w261, "Strings []"=w260) -> ()  [unwired: 2 in, 2 out]
                n164 = property on="Test Ring" class="Ring (strict)"("Visible"=TRUE) -> ()  [unwired: 2 in, 2 out]
                n165 = property on="Test Slider" class="Slide (strict)"("Visible"=FALSE) -> ()  [unwired: 2 in, 2 out]
              }
              frame "Exposure Priority  **" {
                n166 = Index Array(array=w272, index=3) -> (element=w273:cluster{string[]})
                n167 = call <vilib>:"NT Read String.vi"("Name"=w275) -> ("String"=w274:string)  [unwired: 9 in, 1 out]
                n168 = Unbundle(w273) -> (w269:string[])
                n169 = Match First String(2:w269, 3:w274) -> (0:w270:i32)  [unwired: 1 out]
                n170 = property on="Test Ring" class="Ring (strict)"("Value"=w270, "Strings []"=w269) -> ()  [unwired: 2 in, 2 out]
                n171 = property on="Test Ring" class="Ring (strict)"("Visible"=TRUE) -> ()  [unwired: 2 in, 2 out]
                n172 = property on="Test Slider" class="Slide (strict)"("Visible"=FALSE) -> ()  [unwired: 2 in, 2 out]
              }
              frame "Color Enable  **" {
                n173 = Index Array(array=w281, index=4) -> (element=w282:cluster{string[]})
                n174 = call <vilib>:"NT Read String.vi"("Name"=w284) -> ("String"=w283:string)  [unwired: 9 in, 1 out]
                n175 = Unbundle(w282) -> (w278:string[])
                n176 = Match First String(2:w278, 3:w283) -> (0:w279:i32)  [unwired: 1 out]
                n177 = property on="Test Ring" class="Ring (strict)"("Value"=w279, "Strings []"=w278) -> ()  [unwired: 2 in, 2 out]
                n178 = property on="Test Ring" class="Ring (strict)"("Visible"=TRUE) -> ()  [unwired: 2 in, 2 out]
                n179 = property on="Test Slider" class="Slide (strict)"("Visible"=FALSE) -> ()  [unwired: 2 in, 2 out]
              }
              frame Default {
                n180 = property on="Test Ring" class="Ring (strict)"("Visible"=FALSE) -> ()  [unwired: 2 in, 2 out]
                n181 = property on="Test Slider" class="Slide (strict)"("Visible"=FALSE) -> ()  [unwired: 2 in, 2 out]
              }
              frame "Brightness  **", "Color Level  **", "Compression  **", "FPS  **", "Sharpness  **" {
                n182 = call <vilib>:"NT Read Number.vi"("Name"=w290) -> ("Numeric"=w289:dbl)  [unwired: 9 in, 1 out]
                n183 = local write "Test Slider"(w289) -> ()
                n184 = property on="Test Ring" class="Ring (strict)"("Visible"=FALSE) -> ()  [unwired: 2 in, 2 out]
                n185 = property on="Test Slider" class="Slide (strict)"("Visible"=TRUE, "Scale.Maximum"=100.0 ("Scale.Range:Maximum")) -> ()  [unwired: 2 in, 2 out]
              }
            }
          }
        }
        n186 = property on="Progress" class="Clust (strict)"("Visible"=FALSE) -> ()  [unwired: 2 in, 2 out]
      }
      event "Test Name": Mouse Enter {
        # "Populate the ring with the list of tests"
        n187 = event-data() -> ()  [unwired: 1 in, 1 out]
        n188 = call <vilib>:"NT Read String Array.vi"("Name"="TestMode/TestList") -> ("String Array"=w298:string[])  [unwired: 9 in, 1 out]
        n189 = Build Array (concatenate)("Select the test to run...", w298) -> (w297:string[])
        n190 = property on="Test Name" class="Ring (strict)"("Strings []"=w297) -> ()  [unwired: 2 in, 2 out]
      }
      event "Test Name": Value Change {
        w300 = FALSE ("Visible")
        # "Tell the robot the test name to run"
        n191 = event-data() -> ("NewVal"=w304:u16)  [unwired: 1 in]
        n192 = property on="Test Name" class="Ring (strict)"() -> ("Strings []"=w305:string[])  [unwired: 2 in, 2 out]
        n193 = local write "Progress"(T4 {"Test Progress"=0, "Test Progress Text"=""} ("Progress")) -> ()
        n194 = Index Array(array=w305, index=w304) -> (element=w303:string)
        n195 = call <vilib>:"NT Write String.vi"("String"=w303, "Name"="TestMode/TestName") -> ()  [unwired: 9 in, 1 out]
        n196 = property on="Progress" class="Clust (strict)"("Visible"=TRUE) -> ()  [unwired: 2 in, 2 out]
        n197 = property on="Motor" class="Clust (strict)"("Visible"=w300) -> ()  [unwired: 2 in, 2 out]
        n198 = property on="Test Slider" class="Slide (strict)"("Visible"=w300) -> ()  [unwired: 2 in, 2 out]
        n199 = property on="On/Off" class="Bool (strict)"("Visible"=w300) -> ()  [unwired: 2 in, 2 out]
        n200 = property on="Rev/Fwd" class="Clust (strict)"("Visible"=w300) -> ()  [unwired: 2 in, 2 out]
        n201 = property on="Test Ring" class="Ring (strict)"("Visible"=w300) -> ()  [unwired: 2 in, 2 out]
      }
      event "Listbox": Double Click {
        # "Shift clears all"
        # "Update symbols on the listbox"
        n202 = event-data() -> ("PlatMods.Shift"=w308:bool, "Row"=w310:i32)  [unwired: 1 in]
        n203 = case shown="True" w308 {
          tunnel: w310 -> [w314 _]
          tunnel: 1 -> [w313 _]
          frame False {
            n204 = property on="Listbox" class="LstBox (strict)"() -> ("Item Symbols"=w312:i32[])  [unwired: 2 in, 2 out]
            n205 = Replace Array Subset(array=w312, new element=w313, index=w314) -> (w311:i32[])
            n206 = property on="Listbox" class="LstBox (strict)"("Item Symbols"=w311) -> ()  [unwired: 2 in, 2 out]
          }
          frame True {
            w315 = 0 ("Top Row")
            n207 = property on="Listbox" class="LstBox (strict)"() -> ("Number of Rows"=w317:u32)  [unwired: 2 in, 2 out]
            n208 = Initialize Array(0, w317) -> (w316:i32[])
            n209 = property on="Listbox" class="LstBox (strict)"("Top Row"=w315, "Value"=w315, "Item Symbols"=w316) -> ()  [unwired: 2 in, 2 out]
          }
        }
      }
      event "Listbox": Key Down {
        # "Update symbols on the listbox\nLeft and right keys check and uncheck"
        n210 = event-data() -> ("VKey"=w321:T15)  [unwired: 1 in]
        n211 = case shown="\"Left\", \"Right\"" w321 {
          selector: w321 -> [w326 _]
          tunnel: eventvkey."Left" ("VKey") -> [w324 _]
          frame "Left", "Right" {
            n212 = Equal?(x=w324, y=w326) -> (x = y?=w325:bool)
            n213 = Select(t=0, s=w325, f=1) -> (s? t:f=w327:i32)
            n214 = property on="Listbox" class="LstBox (strict)"() -> ("Item Symbols"=w330:i32[])  [unwired: 2 in, 2 out]
            n215 = Replace Array Subset(array=w330, new element=w327, index="Listbox") -> (w329:i32[])
            n216 = property on="Listbox" class="LstBox (strict)"("Item Symbols"=w329) -> ()  [unwired: 2 in, 2 out]
          }
          frame Default {
          }
        }
      }
      event "DB Camera Config": Value Change {
        # "Show or hide the cluster of controls, store in ini file"
        n217 = event-data() -> ("NewVal"=w334:bool)  [unwired: 1 in]
        n218 = case shown="False" w334 {
          tunnel: w333 -> [w343 _]
          tunnel: [w336 w354] -> w332
          tunnel: w331 -> [w335 w354]
          frame False {
            w350 = "Camera"
            w353 = FALSE ("Visible")
            n219 = local read "Camera Settings"() -> (w342:T2)
            n220 = Index Array(array=w343) -> (element=w346:cluster{string[]})  [unwired: 1 in]
            n221 = Unbundle(w342) -> ("Frame Rate"=w341:i32, "Compression"=w340:i32, "Size"=w344:u16)
            n222 = Unbundle(w346) -> (w345:string[])
            n223 = Index Array(array=w345, index=w344) -> (element=w339:string)
            n224 = call-poly <vilib>:"Write Key.vi"("section"=w350, "value"=w339, "key"="Size", "refnum"=w335) -> ("refnum out"=w352:T13)  [unwired: 2 in, 5 out]
            n225 = call-poly <vilib>:"Write Key.vi"("section"=w350, "value"=w341, "key"="FrameRate", "refnum"=w352) -> ("refnum out"=w351:T13)  [unwired: 1 in, 6 out]
            n226 = property on="Camera Settings" class="Clust (strict)"("Visible"=w353) -> ()  [unwired: 2 in, 2 out]
            n227 = local write "DB Camera Config"(w353) -> ()
            n228 = call-poly <vilib>:"Write Key.vi"("section"=w350, "value"=w340, "key"="Compression", "refnum"=w351) -> ("refnum out"=w337:T13)  [unwired: 1 in, 6 out]
            n229 = call <vilib>:"Close Config Data.vi"("refnum"=w337) -> ("file path"=w338:path)  [unwired: 2 in, 8 out]
            n230 = call <vilib>:"Open Config Data.vi"("configuration file path"=w338) -> ("refnum"=w336:T13)  [unwired: 8 in, 2 out]
          }
          frame True {
            n231 = property on="Camera Settings" class="Clust (strict)"("Visible"=TRUE) -> ()  [unwired: 2 in, 2 out]
          }
        }
      }
      event "Camera Settings": Value Change {
        # "Update summary string when any elements of DB camera change"
        n232 = event-data() -> ("NewVal"=w367:T2)  [unwired: 1 in]
        n233 = Index Array(array=w363) -> (element=w362:cluster{string[]})  [unwired: 1 in]
        n234 = Unbundle(w367) -> ("Frame Rate"=w358:i32, "Compression"=w357:i32, "Size"=w360:u16)
        n235 = Unbundle(w362) -> (w361:string[])
        n236 = Index Array(array=w361, index=w360) -> (element=w359:string)
        n237 = Format Into String(format string="%s   %dfps   %d%%", w359, w358, w357) -> (resulting string=w364:string)  [unwired: 2 in, 1 out]
        n238 = Build Array(w364) -> (w365:string[])
        n239 = property on="DB Camera Config" class="Bool (strict)"("Strings [4]"=w365) -> ()  [unwired: 2 in, 2 out]
      }
      event "Motor.Enable": Value Change {
        # "When the test mode otor enable helper is set, update that\ntree row item's value"
        n240 = event-data() -> ("NewVal"=w373:bool)  [unwired: 1 in]
        n241 = Unbundle("Motor") -> ("Value"=w372:dbl)  [unwired: 1 out]
        n242 = Select(t=w372, s=w373, f=0.0) -> (s? t:f=w370:dbl)
        n243 = call <vilib>:"NT Write Number.vi"("Numeric"=w370, "Name"=w369) -> ()  [unwired: 9 in, 1 out]
      }
      event "Test Slider": Value Change {
        # "When the test mode slider helper is set, update that\ntree row item's value"
        n244 = event-data() -> ("NewVal"=w376:dbl)  [unwired: 1 in]
        n245 = call <vilib>:"NT Write Number.vi"("Numeric"=w376, "Name"=w377) -> ()  [unwired: 9 in, 1 out]
      }
      event "On/Off": Value Change {
        # "When the test mode on/off helper value is set, update that\ntree row item's value"
        n246 = event-data() -> ("NewVal"=w381:bool)  [unwired: 1 in]
        n247 = Boolean To (0,1)(Boolean=w381) -> (0, 1=w380:i16)
        n248 = call <vilib>:"NT Write Number.vi"("Numeric"=w380, "Name"=w379) -> ()  [unwired: 9 in, 1 out]
      }
      event "Rev/Fwd": Value Change {
        # "When the test mode helper value for relays is set, update that\ntree row item's value"
        n249 = event-data() -> ("NewVal.Forward"=w389:bool, "NewVal.Reverse"=w388:bool)  [unwired: 1 in]
        n250 = Boolean To (0,1)(Boolean=w389) -> (0, 1=w385:i16)
        n251 = Boolean To (0,1)(Boolean=w388) -> (0, 1=w387:i16)
        n252 = Negate(x=w387) -> (-x=w386:i16)
        n253 = Add(x=w385, y=w386) -> (x+y=w384:i16)
        n254 = call <vilib>:"NT Write Number.vi"("Numeric"=w384, "Name"=w383) -> ()  [unwired: 9 in, 1 out]
      }
      event "Test Ring": Value Change {
        # "When a test mode helper value is selected from the ring,\nset the tree item's variable to the string value"
        n255 = event-data() -> ("NewVal"=w393:u16)  [unwired: 1 in]
        n256 = property on="Test Ring" class="Ring (strict)"() -> ("Strings []"=w394:string[])  [unwired: 2 in, 2 out]
        n257 = Index Array(array=w394, index=w393) -> (element=w392:string)
        n258 = call <vilib>:"NT Write String.vi"("String"=w392, "Name"=w391) -> ()  [unwired: 9 in, 1 out]
      }
      event "Rec Mode": Value Change {
        # "Update globals for recording mode and path to read log from.\nClear when logging and let NetworkTables set path for vision to\nuse."
        n259 = event-data() -> ("NewVal"=w404:enum32{"Stop", "Record", "Playback"})  [unwired: 1 in]
        n260 = case shown="\"Playback\"" w404 {
          tunnel: w403 -> [_ w406 w414]
          tunnel: [_ _ w413] -> w400
          tunnel: [_ _ w412] -> _
          tunnel: w398 -> [_ _ w410]
          tunnel: cluster{i32, i32} {-250, 170} -> [_ _ w409]
          tunnel: [_ _ T16 {"Image Size"=TRUE, "Image Type"=TRUE, "Pixel Value"=TRUE, "ROI Information"=TRUE, "Zoom Factor"=FALSE} ("Image Information Shown:All Elements")] -> w396
          tunnel: [_ _ TRUE ("Zoom Factor")] -> w395
          frame Default {
          }
          frame "Stop", "Record" {
            # "Place Window too"
            n261 = invoke class="VI" method="FP.Close"(reference=w406) -> (reference out=w405:refnum<vi>)  [unwired: 2 in, 2 out]
            n262 = invoke class="VI" method="Abort VI"(reference=w405) -> ()  [unwired: 2 in, 3 out]
          }
          frame "Playback" {
            n263 = call "Open Playback Panel.vi"("Offset"=w409, "DB VI Ref"=w410, "Playback in"=w414) -> ("Playback out"=w411:refnum<vi>)  [unwired: 8 in]
            n264 = register-events(w411) -> (reference out=w413:refnum<event-registration>, error out=w412:errorcluster)  [unwired: 2 in]
          }
        }
        n265 = global write "WPI_DashboardLogging Global.vi" "Recording"(w404) -> ()
        n266 = global write "WPI_DashboardLogging Global.vi" "Logging Filename"(path "") -> ()
        n267 = property on="Camera Image" class="ImageControl"("Image Information Shown"=w396, "Image Information Visible"=w395) -> ()  [unwired: 2 in, 2 out]
        n268 = call <vilib>:"WPI_DashboardNT Log FieldName Cache.vi"("Operation"=enum16{"Lookup/Add", "Index", "Clear"}."Clear") -> ()  [unwired: 8 in, 3 out]
      }
      event Panel Close {
        w415 = enum32{"Stop", "Record", "Playback"}."Stop" ("Rec Mode")
        # "Playback window has been closed, abort"
        n269 = event-data() -> ()  [unwired: 1 in, 4 out]
        n270 = local write "Rec Mode"(w415) -> ()
        n271 = global write "WPI_DashboardLogging Global.vi" "Recording"(w415) -> ()
      }
      event Panel Close {
        # "Abort playback window and ourself"
        n272 = event-data() -> ()  [unwired: 1 in, 4 out]
        n273 = invoke class="VI" method="FP.Close"(reference=w420) -> (reference out=w419:refnum<vi>)  [unwired: 2 in, 2 out]
        n274 = invoke class="VI" method="Abort VI"(reference=w419) -> (error out=w418:errorcluster)  [unwired: 2 in, 2 out]
        n275 = invoke class="VI" method="Abort VI"(error in=w418) -> ()  [unwired: 2 in, 3 out]
      }
      event "Vision": Value Change {
        # "Enable/Disable Compression slider.\nHW USB is hard-coded into the camera"
        n276 = event-data() -> ("NewVal"=w426:u16)  [unwired: 1 in]
        n277 = Equal?(x=w426, y=u32 2 ("milliseconds to wait")) -> (x = y?=w424:bool)
        n278 = Select(t=T17."Disabled and Grayed Out" ("Disabled"), s=w424, f=T17."Enabled" ("Disabled")) -> (s? t:f=w421:T17)
        n279 = property on="Compression" class="Slide (strict)"("DisabledEnum"=w421) -> ()  [unwired: 2 in, 2 out]
      }
    }
  }
  n280 = while {
    tunnel: w38 -> [w429]
    i -> [w432]
    stop <- FALSE stop-if-true
    n281 = Wait (ms)(milliseconds to wait=u32 100) -> ()  [unwired: 1 out]
    n282 = case shown="\"Playback\"" "Rec Mode" {
      tunnel: w432 -> [_ _ w447]
      tunnel: [u32 2829099 ("Base Color") u32 11141120 ("Target Color") w436] -> w428
      frame "Stop", Default {
        # "Reset the color, extra updates don't cost much"
      }
      frame "Record" {
      }
      frame "Playback" {
        # "Playback"
        n283 = Quotient & Remainder(x=w447, y=u32 50 ("milliseconds to wait")) -> (x-y*floor(x/y)=w443:u32)  [unwired: 1 out]
        n284 = Divide(x=w443, y=u32 50 ("milliseconds to wait")) -> (x/y=w440:dbl)
        n285 = Multiply(x=6.283185307179586, y=w440) -> (x*y=w445:dbl)
        n286 = Sine(x=w445) -> (sin(x)=w444:dbl)
        n287 = Absolute Value(x=w444) -> (abs(x)=w437:dbl)
        n288 = call "Interpolate RGB Color.vi"("Proportion"=w437, "Target Color"=u32 30976, "Base Color"=u32 2829099) -> ("Result Color"=w436:u32)  [unwired: 8 in]
      }
    }
    n289 = property class="Pane"(reference=w429, "PaneColor"=w428) -> ()  [unwired: 1 in, 2 out]
  }
  n290 = TCP Create Listener(10:u16 1741 ("timeout ms (25000)")) -> (3:w1:refnum<k5>)  [unwired: 4 in, 2 out]
  n291 = while {
    tunnel: w1 -> [w449]
    stop <- FALSE stop-if-true
    n292 = TCP Wait On Listener(11:w449) -> (4:w448:refnum<k5>)  [unwired: 3 in, 4 out]
    n293 = local write "TCP"(w448) -> ()
  }
  n294 = property on="On/Off" class="Bool (strict)"("Visible"=w6) -> ()  [unwired: 2 in, 2 out]
  n295 = property on="Motor" class="Clust (strict)"("Visible"=w6) -> ()  [unwired: 2 in, 2 out]
  n296 = property on="Progress" class="Clust (strict)"("Visible"=w6) -> ()  [unwired: 2 in, 2 out]
  n297 = property on="Test Ring" class="Ring (strict)"("Visible"=w6) -> ()  [unwired: 2 in, 2 out]
  n298 = property on="Rev/Fwd" class="Clust (strict)"("Visible"=w6) -> ()  [unwired: 2 in, 2 out]
  n299 = property on="Camera Settings" class="Clust (strict)"("Visible"=w6) -> ()  [unwired: 2 in, 2 out]
  n300 = local write "DB Camera Config"(w6) -> ()
  n301 = global write "WPI_DashboardLogging Global.vi" "Recording"(w32) -> ()
  n302 = local write "Rec Mode"(w32) -> ()
